vi "Set Report Font.vi"(0 "report in":refnum<class "ooCalc.lvclass">, 1 "text color (unchanged)":u32(colorbox)=16777216, 2 "font settings source":u16(ring) items=["VI Inputs", "Font Dialog Box"], 5 "text options":T2, 9 "font settings":T3={"Charset (-1)"=-1, "Weight (-1)"=-1, "Name"="", "Size"=" "}, 11 "error in (no error)":errorcluster) -> (4 "report out":refnum<class "ooCalc.lvclass">, 6 "font out":T1={"font name"="", "font size"=0.0, "bold"=0, "italic"=0, "underline"=0, "strike through"=0, "font color"=16777216} {"font size" format="%0.2f"; "strike through" items=["Unchanged", "Yes", "No"]; "underline" items=["Unchanged", "Yes", "No"]; "italic" items=["Unchanged", "Yes", "No"]; "bold" items=["Unchanged", "Yes", "No"]}, 15 "error out":errorcluster)   [LabVIEW 2009, in "ooCalc.lvclass"]
doc: "Sets the font properties of the report, including those in the headers and footers."
uses:
  ooCalc.lvclass
  <vilib>/Utility/NIReport.llb/font.ctl
  ooCalc.lvclass/ooCalc.ctl
  C:/Projets/LAVAG/OpenOfficeRGT/AODL/DLLs/AODL.dll
  <vilib>/Utility/NIReport.llb/NI_ReportGenerationCore.lvlib
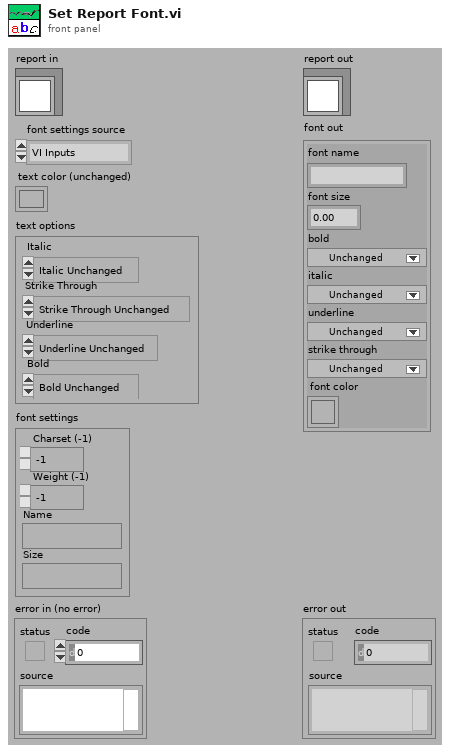
[diagram p1: front panel]
types:
  T1 = typedef "NI_ReportGenerationCore.lvlib/font.ctl" = cluster{"font name":string, "font size":dbl, "bold":u16, "italic":u16, "underline":u16, "strike through":u16, "font color":u32}
  T2 = cluster{"Italic":enum16{"Italic Unchanged", "Italic On", "Italic Off"}, "Strike Through":enum16{"Strike Through Unchanged", "Strike Through On", "Strike Through Off"}, "Underline":enum16{"Underline Unchanged", "Underline On", "Underline Off"}, "Bold":enum16{"Bold Unchanged", "Bold On", "Bold Off"}}
  T3 = cluster{"Charset (-1)":i16, "Weight (-1)":i16, "Name":string, "Size":string}
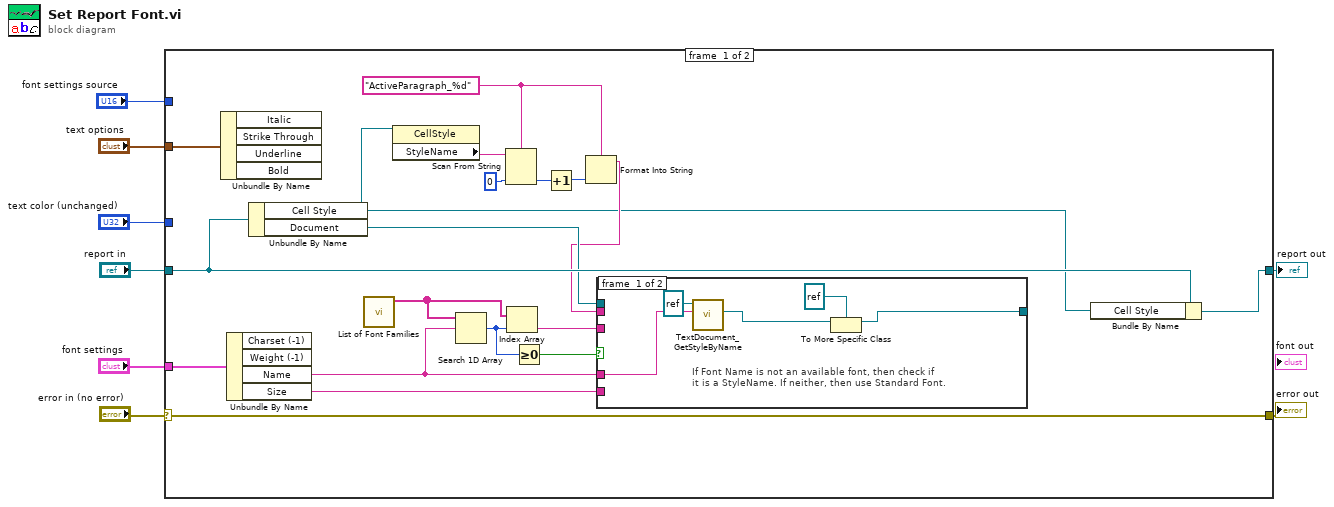
[diagram p0: block diagram]
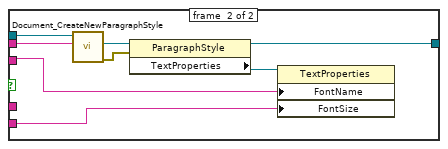
[diagram p2: hidden frame]
diagram:
  n1 = case shown="No Error" "error in (no error)" {
    selector: "error in (no error)" -> [w27 w41]
    tunnel: [w27 w41] -> w8
    tunnel: "report in" -> [w19 w42]
    tunnel: [w18 w42] -> w6
    tunnel: "font settings" -> [w25 _]
    tunnel: "text options" -> [w26 _]
    tunnel: "text color (unchanged)" -> [_ _]
    tunnel: "font settings source" -> [_ _]
    frame #0 {
      w20 = "ActiveParagraph_%d" ("styleName")
      n2 = Unbundle By Name(w26) -> ()  [unwired: 4 out]
      n3 = Unbundle By Name(w25) -> ("Name"=w10:string, "Size"=w11:string)  [unwired: 2 out]
      n4 = Unbundle By Name(w19) -> ("Cell Style"=w9:refnum<k24>, "Document"=w14:refnum<k24>)
      n5 = call "List of Font Families.vi"() -> ("Available Fonts"=w17:string[])  [unwired: 11 in]
      n6 = property class="CellStyle"(reference=w9) -> ("StyleName"=w24:string)  [unwired: 1 in, 2 out]
      n7 = Search 1D Array(1D array=w17, element=w10) -> (index of element=w16:i32)  [unwired: 1 in]
      n8 = Scan From String(format string=w20, input string=w24, default 1=0 ("default value 1")) -> (output 1=w22:i32)  [unwired: 2 in, 3 out]
      n9 = Index Array(array=w17, index=w16) -> (element=w12:string)
      n10 = Greater Or Equal To 0?(x=w16) -> (x >= 0?=w15:bool)
      n11 = Increment(x=w22) -> (x+1=w21:i32)
      n12 = Format Into String(format string=w20, w21) -> (resulting string=w13:string)  [unwired: 2 in, 1 out]
      n13 = case shown="False" w15 {
        tunnel: w14 -> [_ w40]
        tunnel: [w30 w33] -> _
        tunnel: w13 -> [_ w39]
        tunnel: w12 -> [_ w35]
        tunnel: w11 -> [_ w34]
        tunnel: w10 -> [w29 _]
        frame #0 {
          # "If Font Name is not an available font, then check if\nit is a StyleName. If neither, then use Standard Font."
          n14 = call "TextDocument_GetStyleByName.vi"("StyleName"=w29, "TextDocument in"=refnum<k24> refnum) -> ("Style"=w32:refnum<k24>)  [unwired: 7 in, 2 out]
          n15 = To More Specific Class(target class=refnum<k24> refnum, reference=w32) -> (specific class reference=w30:refnum<k24>)  [unwired: 1 in, 1 out]
        }
        frame #1 {
          n16 = call "Document_CreateNewParagraphStyle.vi"("styleName"=w39, "document"=w40) -> ("error out"=w37:errorcluster, "Paragraph Style"=w38:refnum<k24>)  [unwired: 7 in, 1 out]
          n17 = property class="ParagraphStyle"(reference=w38, error in=w37) -> (reference out=w33:refnum<k24>, "TextProperties"=w36:refnum<k24>)  [unwired: 1 out]
          n18 = property class="TextProperties"(reference=w36, "FontName"=w35, "FontSize"=w34) -> ()  [unwired: 1 in, 2 out]
        }
      }
      n19 = Bundle By Name(cluster=w19, "Cell Style"=w9) -> (w18:refnum<class "ooCalc.lvclass">)
    }
    frame #1 {
    }
  }
  "error out" <- w8
  "report out" <- w6
